vi "Configure Step.vi"(8 "error in":errorcluster, 9 "Step value(V/A)":dbl min=0.0 format="%.2g", 10 "Type":u16(ring) items=["Voltage", "Current"], 11 "VISA resource name":refnum<visa-resource-name>) -> (0 "error out":errorcluster, 3 "VISA resource name out":refnum<visa-resource-name>)   [LabVIEW 2015, in "IT6700H.lvlib"]
doc: "Sets the step value of the voltage or the current.\n<b>Type</b>\n0: Voltage\n1: Current\n<b>Step Value(V/A)</b>\n0-MAX"
uses:
  <instrlib>/IT6700H/IT6700H.lvlib
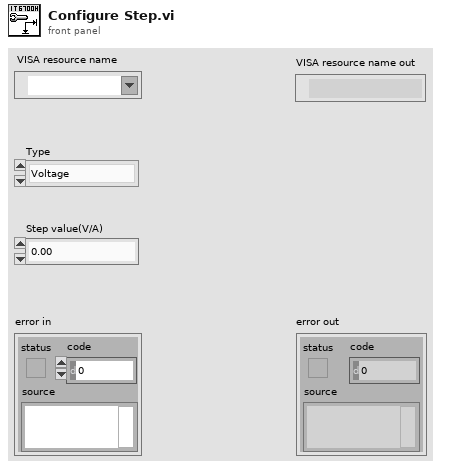
[diagram p1: front panel]
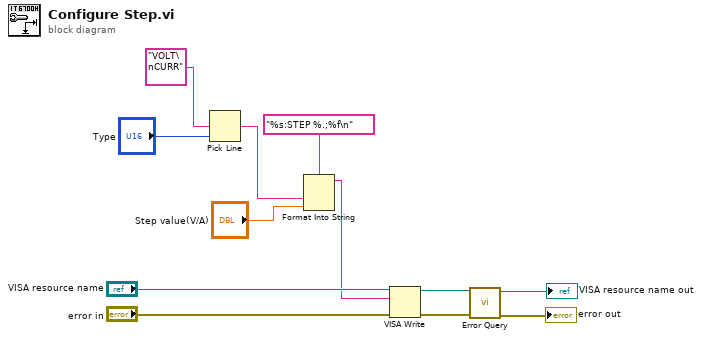
[diagram p0: block diagram]
diagram:
  n1 = Pick Line(multi-line string="VOLT\nCURR", line index="Type") -> (output string=w8:string)  [unwired: 1 in]
  n2 = Format Into String(format string="%s:STEP %.;%f\n", w8, "Step value(V/A)") -> (resulting string=w5:string)  [unwired: 2 in, 1 out]
  n3 = VISA Write(VISA resource name="VISA resource name", write buffer=w5, error in (no error)="error in") -> (VISA resource name out=w3:refnum<visa-resource-name>, error out=w4:errorcluster)  [unwired: 1 out]
  n4 = call <instrlib>:"Error Query.vi"("error in"=w4, "VISA resource name"=w3) -> ("error out"=→"error out":errorcluster, "VISA resource name out"=→"VISA resource name out":refnum<visa-resource-name>)  [unwired: 6 in, 2 out]
